vi "Data Server.vi"() -> ()   [LabVIEW 2010]
doc: "Sends a specified waveform through a TCP port. The VI first listens for a connection and, once established, sends the number of bytes to be sent followed by the data. After the data is sent, the VI waits for an 'all received' signal from the client and then breaks the connection.\n\n<B>Note:</B> Requires the Data Client.vi located in the same library as this VI."
panel:
  in  "stop":bool
  in  "Port":u16=6340 min=1025 step=1
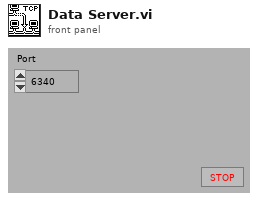
[diagram p1: front panel]
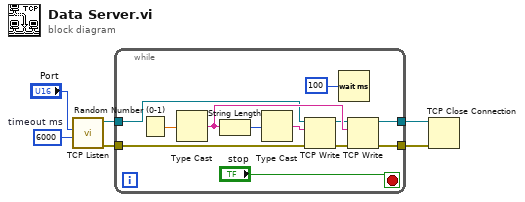
[diagram p0: block diagram]
diagram:
  w4 = 6000  # timeout ms
  n1 = call <vilib>:"TCP Listen.vi"("timeout ms (wait forever: -1)"=w4, "port"="Port") -> ("error out"=w6:errorcluster, "connection ID"=w2:refnum<k5>)  [unwired: 6 in, 2 out]
  n2 = while {
    tunnel: w6 -> [w13]
    tunnel: [w9] -> w3
    tunnel: w2 -> [w8]
    tunnel: [w7] -> w1
    stop <- "stop" stop-if-true
    n3 = Random Number (0-1)() -> (number: 0 to 1=w14:dbl)
    n4 = Type Cast(x=w14) -> (*(type *) &x=w18:string)  [unwired: 1 in]
    n5 = String Length(string=w18) -> (length=w16:i32)
    n6 = Type Cast(x=w16) -> (*(type *) &x=w17:string)  [unwired: 1 in]
    n7 = TCP Write(connection ID=w8, data in=w17, error in (no error)=w13) -> (connection ID out=w15:refnum<k5>, error out=w12:errorcluster)  [unwired: 1 in, 1 out]
    n8 = Wait (ms)(milliseconds to wait=u32 100) -> ()  [unwired: 1 out]
    n9 = TCP Write(connection ID=w15, data in=w18, error in (no error)=w12) -> (connection ID out=w7:refnum<k5>, error out=w9:errorcluster)  [unwired: 1 in, 1 out]
  }
  n10 = TCP Close Connection(connection ID=w1, error in (no error)=w3) -> ()  [unwired: 1 in, 2 out]
